vi "pixToStr.vi"(11 "Disabled Pixels":u8[](array[numeric])) -> (3 "Disabled pixels string":string)   [LabVIEW 2018]
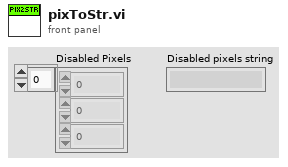
[diagram p1: front panel]
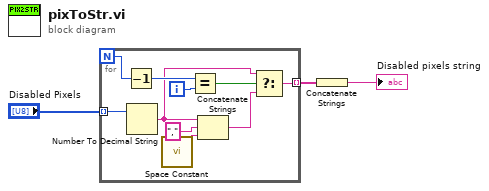
[diagram p0: block diagram]
diagram:
  n1 = for {
    N -> [w10]
    tunnel: "Disabled Pixels" -> [w12] mode=indexing
    tunnel: [w6] -> w1 mode=indexing
    i -> [w9]
    n2 = Decrement(x=w10) -> (x-1=w8:i32)
    n3 = Number To Decimal String(number=w12) -> (decimal integer string=w7:string)  [unwired: 1 in]
    n4 = call <vilib>:"Space Constant.vi"() -> ("String"=w11:string)
    n5 = Equal?(x=w8, y=w9) -> (x = y?=w4:bool)
    n6 = Concatenate Strings(w7, ",", w11) -> (w5:string)
    n7 = Select(t=w7, s=w4, f=w5) -> (s? t:f=w6:string)
  }
  n8 = Concatenate Strings(w1) -> (→"Disabled pixels string":string)
